vi "usrp find.vi"(8 "error in (no error)":errorcluster, 10 "strings_out":u64, 11 "args":string) -> (0 "error out":errorcluster, 2 "strings_out out":u64, 3 "function return":u32(ring))   [LabVIEW 2023, in "uhd.lvlib"]
doc: "UHD_API uhd_error uhd_usrp_find(const char* args, uhd_string_vector_handle* strings_out);"
uses:
  <userlib>/uhd/uhd.lvlib
  <userlib>/uhd/uhd.dll
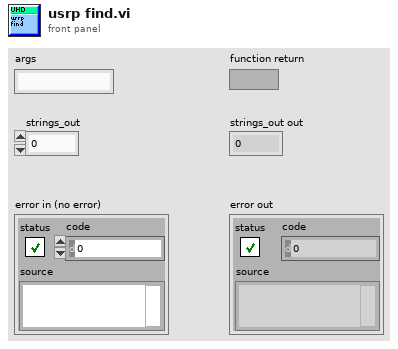
[diagram p1: front panel]
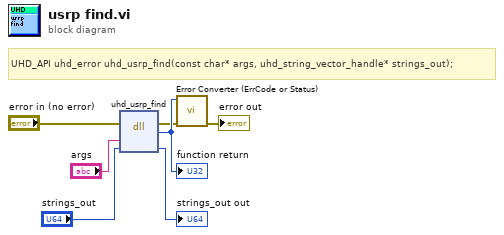
[diagram p0: block diagram]
diagram:
  # "UHD_API uhd_error uhd_usrp_find(const char* args, uhd_string_vector_handle* strings_out);"
  n1 = dll-call lib="C:/Program Files/National Instruments/LabVIEW 2023/user.lib/uhd/uhd.*" fn="uhd_usrp_find"(error in="error in (no error)", "args"="args", "strings_out"="strings_out") -> (error out=w2:errorcluster, w7:u32, "strings_out"=→"strings_out out":u64)  [unwired: 3 in, 1 out]
  "function return" <- w7
  n2 = call <userlib>:"Error Converter (ErrCode or Status).vi"("error in (no error)"=w2, "error code"=w7) -> ("error out"=→"error out":errorcluster)  [unwired: 9 in]
